vi "SendAndRecive.vi"(8 "error in":errorcluster, 9 "Parameters":string, 10 "Command":T2, 11 "connection ID in":refnum<k5>) -> (0 "error out":errorcluster, 1 "Error Info":T1, 2 "Answer":string, 3 "connection ID out":refnum<k5>, 4 "Log String":string)   [LabVIEW 2020, in "ProdigyRemoteControl.lvlib"]
uses:
  ProdigyRemoteControl.lvlib
  DEFINITIONS/DEF_RcCmd.ctl
  DEFINITIONS/DEF_RcError.ctl
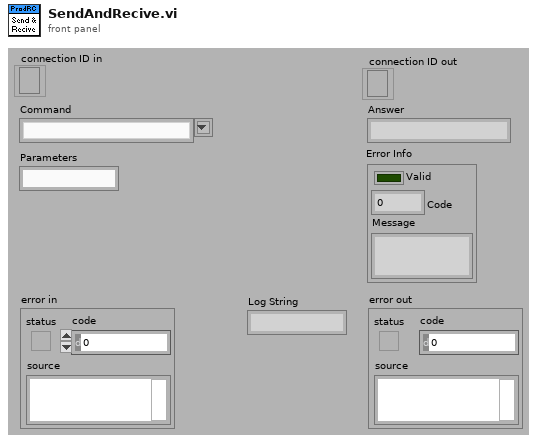
[diagram p1: front panel]
types:
  T1 = typedef "ProdigyRemoteControl.lvlib/DEF_RcError.ctl" = cluster{"Valid":bool, "Code":u16, "Message":string}
  T2 = typedef "ProdigyRemoteControl.lvlib/DEF_RcCmd.ctl" = string
  T3 = enum16{"Standard", "Buffered", "CRLF", "Immediate"}
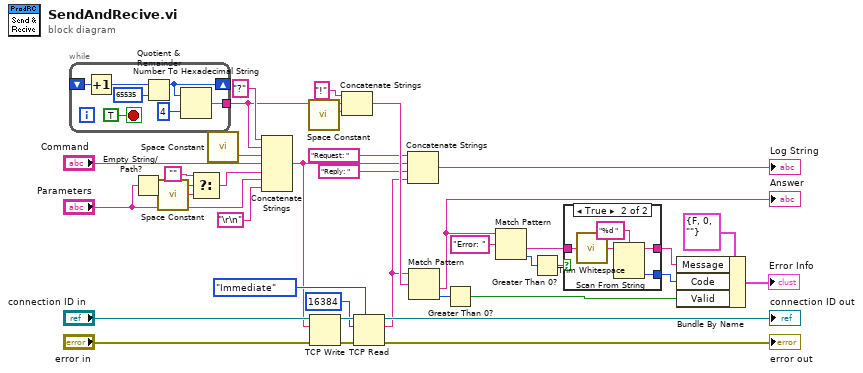
[diagram p0: block diagram]
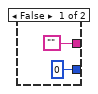
[diagram p2: hidden frame]
diagram:
  n1 = while {
    shift-right: [w38] -> _
    shift-left: _ -> [w44]
    tunnel: [w39] -> w22
    stop <- TRUE stop-if-true
    n2 = Increment(x=w44) -> (x+1=w43:i32)
    n3 = Quotient & Remainder(x=w43, y=65535) -> (x-y*floor(x/y)=w38:i32)  [unwired: 1 out]
    n4 = Number To Hexadecimal String(1:i16 4 ("width (-)"), 2:w38) -> (0:w39:string)
  }
  n5 = Empty String/Path?(string/path="Parameters") -> (empty?=w27:bool)
  n6 = call <vilib>:"Space Constant.vi"() -> ("String"=w25:string)
  n7 = Select(t="", s=w27, f=w25) -> (s? t:f=w24:string)
  n8 = call <vilib>:"Space Constant.vi"() -> ("String"=w18:string)
  n9 = Concatenate Strings("?" ("string"), w22, w18, "Command", w24, "Parameters", "\r\n") -> (w14:string)
  n10 = call <vilib>:"Space Constant.vi"() -> ("String"=w21:string)
  n11 = TCP Write(connection ID="connection ID in", data in=w14, error in (no error)="error in") -> (connection ID out=w31:refnum<k5>, error out=w32:errorcluster)  [unwired: 1 in, 1 out]
  n12 = Concatenate Strings("!" ("string"), w22, w21) -> (w20:string)
  n13 = TCP Read(connection ID=w31, bytes to read=16384, error in (no error)=w32, 7:T3."Immediate" ("mode (standard)")) -> (connection ID out=→"connection ID out":refnum<k5>, data out=w12:string, error out=→"error out":errorcluster)  [unwired: 1 in]
  n14 = Concatenate Strings("Request: " ("string"), w14, "Reply: " ("string"), w12) -> (→"Log String":string)
  n15 = Match Pattern(string=w12, regular expression=w20) -> (after substring=w7:string, offset past match=w19:i32)  [unwired: 1 in, 2 out]
  "Answer" <- w7
  n16 = Greater Than 0?(x=w19) -> (x > 0?=w9:bool)
  n17 = Match Pattern(string=w7, regular expression="Error: ") -> (after substring=w4:string, offset past match=w5:i32)  [unwired: 1 in, 2 out]
  n18 = Greater Than 0?(x=w5) -> (x > 0?=w3:bool)
  n19 = case shown="True" w3 {
    tunnel: w4 -> [_ w51]
    tunnel: [0 w48] -> w2
    tunnel: ["" w47] -> w1
    frame False {
    }
    frame True {
      n20 = call <vilib>:"Trim Whitespace.vi"("string"=w51) -> ("trimmed string"=w49:string)  [unwired: 1 in]
      n21 = Scan From String(format string="%d ", input string=w49) -> (remaining string=w47:string, output 1=w48:i32)  [unwired: 3 in, 2 out]
    }
  }
  n22 = Bundle By Name(cluster=T1 {"Valid"=FALSE, "Code"=0, "Message"=""} ("Error Info"), "Message"=w1, "Code"=w2, "Valid"=w9) -> (→"Error Info":T1)
